vi "queue system.vi"(11 "Mode":enum16{"Get Queue", "New Queue"}(ring)) -> ()   [LabVIEW 2013]
uses:
  typedefs/queue typedef.ctl
  <vilib>/Rock Robotics/WPI/Solenoid/WPI_SolenoidValue.ctl
panel:
  in  "Queue Type":enum16{"Cock", "Uncock", "Shoot"}(ring)
  # "Queue all the things!"
  # "The pneumatics"
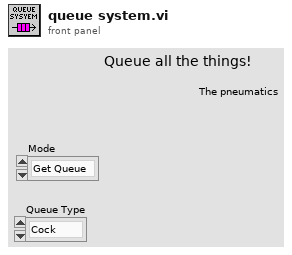
[diagram p1: front panel]
types:
  T1 = typedef "queue typedef.ctl" = cluster{"Pistons":enum16{"Shooter", "Latch"}, "Value":T2, "Wait?":bool, "Wait Time":u16}
  T2 = typedef "WPI_SolenoidValue.ctl" = enum16{"Off", "On", "Forward", "Reverse"}
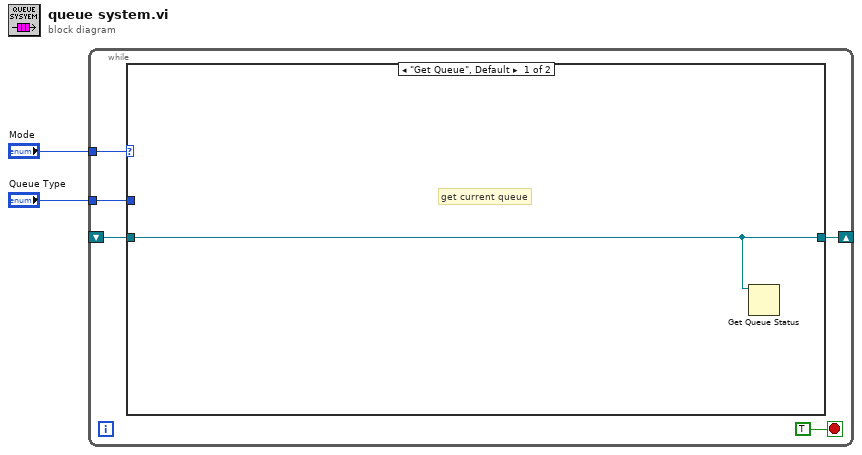
[diagram p0: block diagram]
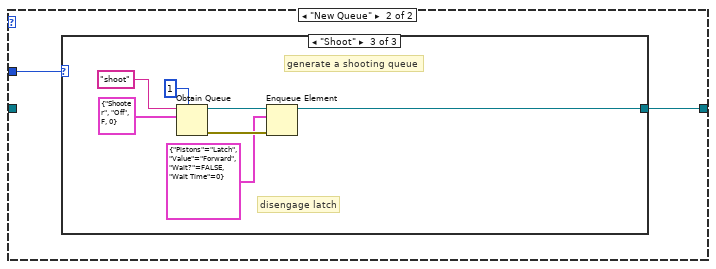
[diagram p2: hidden frame]
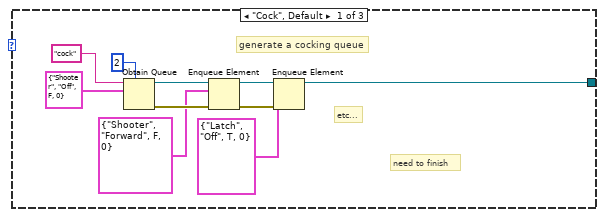
[diagram p3: hidden frame]
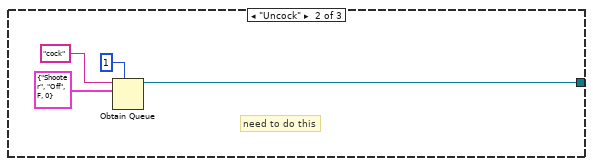
[diagram p4: hidden frame]
diagram:
  n1 = while {
    tunnel: "Mode" -> [w6]
    tunnel: "Queue Type" -> [w5]
    shift-right: [w4] -> _
    shift-left: _ -> [w3]
    stop <- TRUE stop-if-true
    n2 = case shown="\"Get Queue\", Default" w6 {
      tunnel: w5 -> [_ w10]
      tunnel: [w8 w9] -> w4
      tunnel: w3 -> [w8 _]
      frame "Get Queue", Default {
        # "get current queue"
        n3 = Get Queue Status(queue=w8) -> ()  [unwired: 2 in, 8 out]
      }
      frame "New Queue" {
        n4 = case shown="\"Shoot\"" w10 {
          tunnel: [w11 w21 w25] -> w9
          frame "Cock", Default {
            # "need to finish"
            # "etc..."
            # "generate a cocking queue"
            n5 = Obtain Queue(max queue size (-1, unlimited)=2, name (unnamed)="cock", element data type=T1 {"Pistons"=enum."Shooter", "Value"=enum."Off", "Wait?"=FALSE, "Wait Time"=0} ("Queue Datatype")) -> (queue out=w17:refnum<queue>, error out=w16:errorcluster)  [unwired: 2 in, 1 out]
            n6 = Enqueue Element(queue=w17, element=T1 {"Pistons"=enum."Shooter", "Value"=enum."Forward", "Wait?"=FALSE, "Wait Time"=0}, error in (no error)=w16) -> (queue out=w13:refnum<queue>, error out=w14:errorcluster)  [unwired: 1 in, 1 out]
            n7 = Enqueue Element(queue=w13, element=T1 {"Pistons"=enum."Latch", "Value"=enum."Off", "Wait?"=TRUE, "Wait Time"=0}, error in (no error)=w14) -> (queue out=w11:refnum<queue>)  [unwired: 1 in, 2 out]
          }
          frame "Uncock" {
            # "need to do this"
            n8 = Obtain Queue(max queue size (-1, unlimited)=1, name (unnamed)="cock", element data type=T1 {"Pistons"=enum."Shooter", "Value"=enum."Off", "Wait?"=FALSE, "Wait Time"=0} ("Queue Datatype")) -> (queue out=w21:refnum<queue>)  [unwired: 2 in, 2 out]
          }
          frame "Shoot" {
            # "generate a shooting queue"
            # "disengage latch"
            n9 = Obtain Queue(max queue size (-1, unlimited)=1, name (unnamed)="shoot", element data type=T1 {"Pistons"=enum."Shooter", "Value"=enum."Off", "Wait?"=FALSE, "Wait Time"=0} ("Queue Datatype")) -> (queue out=w28:refnum<queue>, error out=w27:errorcluster)  [unwired: 2 in, 1 out]
            n10 = Enqueue Element(queue=w28, element=T1 {"Pistons"=enum."Latch", "Value"=enum."Forward", "Wait?"=FALSE, "Wait Time"=0}, error in (no error)=w27) -> (queue out=w25:refnum<queue>)  [unwired: 1 in, 2 out]
          }
        }
      }
    }
  }
